vi "solar_target.vi"(11 "Target":string) -> ()   [LabVIEW 2018]
doc: "SOLAR target template."
uses:
  solar/solar.lvclass
  solar/solar Msg EnQ (This).vi
  solar/solar Msg UE Generate.vi
  voyager/solar_voy_def/solar_voy_def Import (Variants).vi
  solar/solar Msg Voyager (TLM).vi
panel:
  in  "data in":cluster{dbl}
  out "data out":cluster{dbl}
  out "Time":timestamp
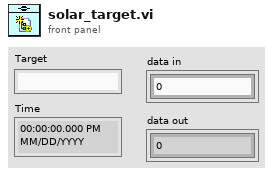
[diagram p1: front panel]
types:
  T1 = typedef "solar_voy_def_ctl PACKET.ctl" = cluster{"PACKET_ID":T2, "ENDIAN":enum8{"BIG", "LITTLE"}, "DESC":string, "HZRD":bool, "ITEMS":T3[], "NoExport":bool, "last_time":timestamp, "last_count":u32, "last_data":string}
  T2 = typedef "solar_voy_def_ctl PACKET_ID.ctl" = cluster{"ID":u16, "CMD":enum8{"CMD", "TLM"}, "TARGET":string, "PACKET":string}
  T3 = typedef "solar_voy_def_ctl ITEM.ctl" = cluster{"NAME":string, "OFFSET":i32, "SIZE":i32, "TYPE":T4, "EACH_SIZE":i32, "LVTYPE":T5, "MIN":dbl, "MAX":dbl, "DEFAULT":string, "DESC":string, "ID":bool, "MODIFIERS":variant, "last_value":variant}
  T4 = typedef "solar_voy_def_ctl ITEM TYPE.ctl" = enum8{"BLOCK", "INT", "UINT", "FLOAT", "STRING"}
  T5 = typedef "solar_type Item Type.ctl" = enum16{"NULL", "UNKNOWN", "CLUSTER", "I8", "I16", "I32", "I64", "U8", "U16", "U32", "U64", "U8_ENUM", "U16_ENUM", "U32_ENUM", "SGL", "DBL", "BOOLEAN", "STRING", "PATH", "VISA", "TAG", "TIME", "I8_1D", "I16_1D", "I32_1D", "I64_1D", "U8_1D", "U16_1D", "U32_1D", "U64_1D", "U8_ENUM_1D", "U16_ENUM_1D", "U32_ENUM_1D", "SGL_1D", "DBL_1D", "BOOLEAN_1D", "STRING_1D", "PATH_1D", "VISA_1D", "TAG_1D", "TIME_1D", "I8_2D", "I16_2D", "I32_2D", "I64_2D", "U8_2D", "U16_2D", "U32_2D", "U64_2D", "U8_ENUM_2D", "U16_ENUM_2D", "U32_ENUM_2D", "SGL_2D", "DBL_2D", "BOOLEAN_2D", "STRING_2D", "PATH_2D", "VISA_2D", "TAG_2D", "TIME_2D"}
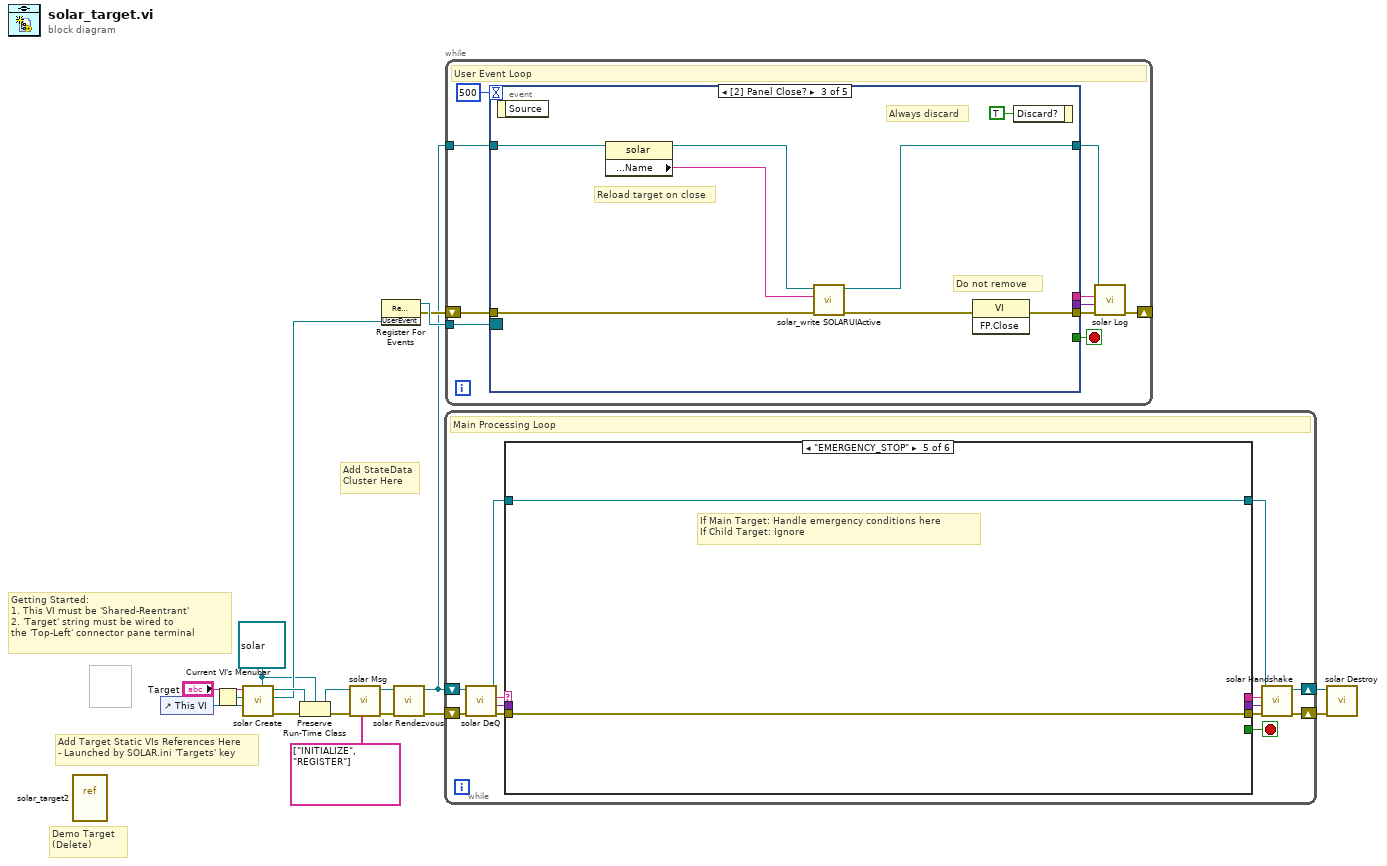
[diagram p0: block diagram]
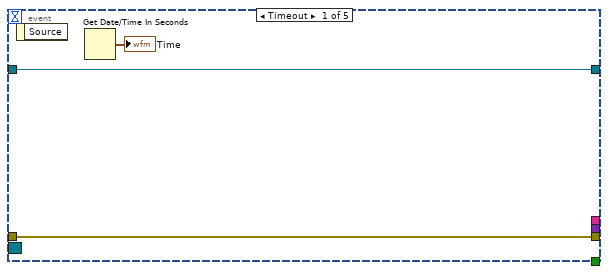
[diagram p2: hidden frame]
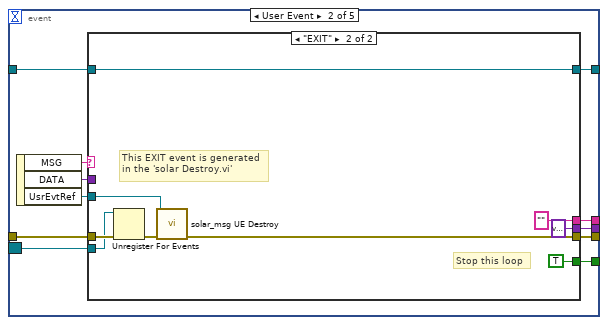
[diagram p3: hidden frame]
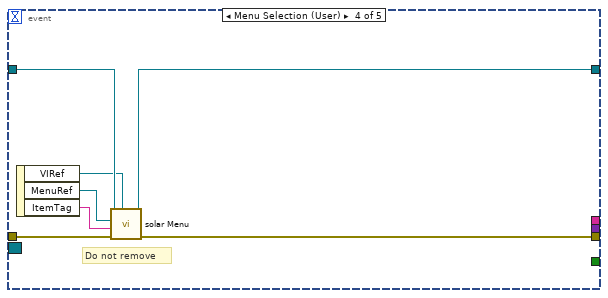
[diagram p5: hidden frame]
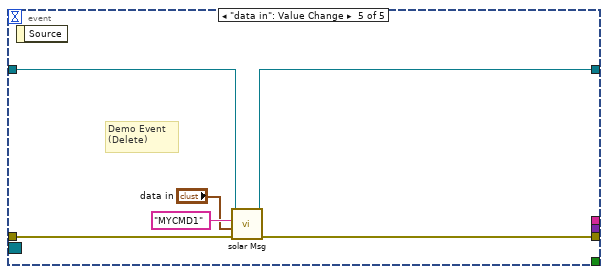
[diagram p6: hidden frame]
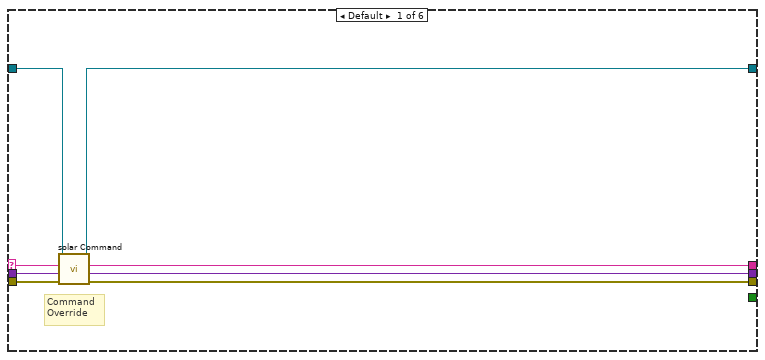
[diagram p7: hidden frame]
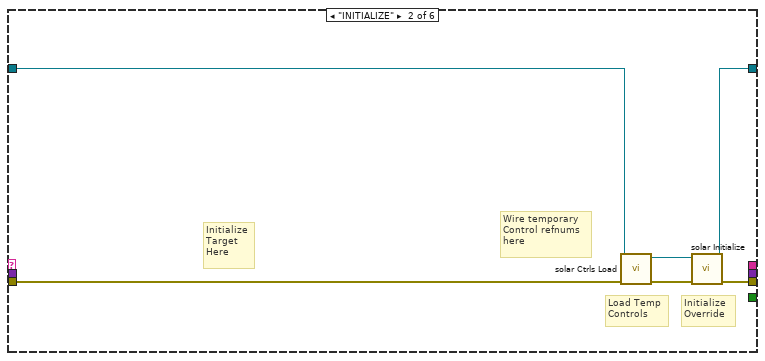
[diagram p8: hidden frame]
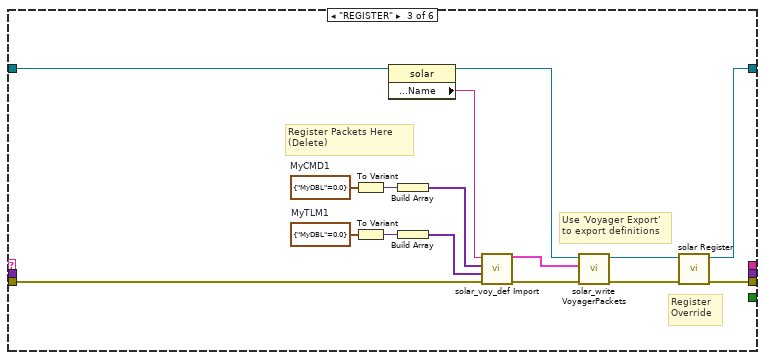
[diagram p9: hidden frame]
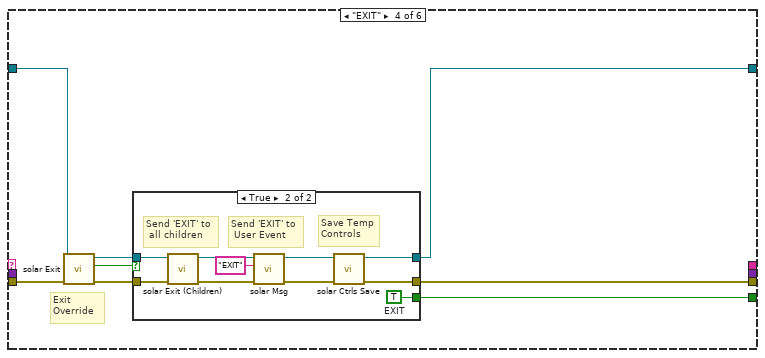
[diagram p10: hidden frame]
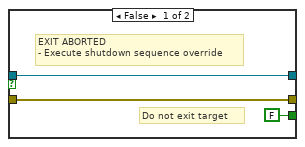
[diagram p11: hidden frame]
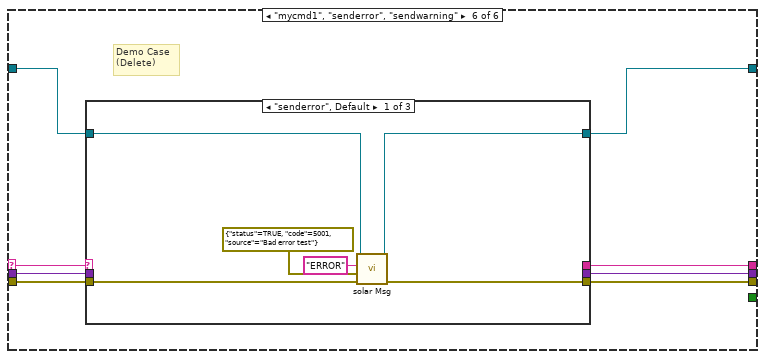
[diagram p12: hidden frame]
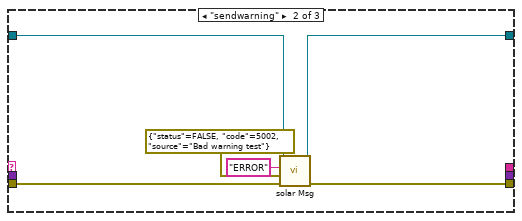
[diagram p13: hidden frame]
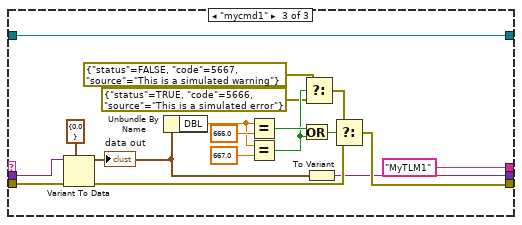
[diagram p14: hidden frame]
diagram:
  w11 = refnum<class "solar.lvclass"> refnum ("Default LVClass")
  # "Demo Target\n(Delete)"
  # "Getting Started:\n1. This VI must be 'Shared-Reentrant'\n2. 'Target' string must be wired to \nthe 'Top-Left' connector pane terminal"
  # "Add StateData\nCluster Here"
  # "Add Target Static VIs References Here\n- Launched by SOLAR.ini 'Targets' key"
  n1 = vi-ref "solar_target2.vi"() -> ()  [unwired: 1 out]
  n2 = control-ref of="This VI"() -> (w13:refnum<vi>)
  n3 = Current VI's Menubar() -> (w9:refnum<k9>)
  n4 = call "solar Create.vi"("Default LVClass"=w11, "VI Refnum"=w13, "VI MenuRef"=w9, "Target"="Target") -> ("error out"=w7:errorcluster, "UserEvent"=w14:refnum<user-event>, "solar"=w18:refnum<class "solar.lvclass">)  [unwired: 4 in, 1 out]
  n5 = Preserve Run-Time Class(object in=w18, error in=w7, 2:w11) -> (object out=w1:refnum<class "solar.lvclass">, error out=w3:errorcluster)
  n6 = call-poly "solar Msg.vi"("MSG Array"=string[] ["INITIALIZE", "REGISTER"] ("Script (\"PACKET{ITEM:VAL}\")"), "error in (no error)"=w3, "solar in"=w1) -> ("error out"=w6:errorcluster, "solar out"=w4:refnum<class "solar.lvclass">)  [unwired: 6 in, 1 out]
  n7 = register-events(w14) -> (reference out=w15:refnum<event-registration>, error out=w8:errorcluster)  [unwired: 2 in]
  n8 = call-dynamic "solar Rendezvous.vi"("error in (no error)"=w6, "solar in"=w4) -> ("error out"=w5:errorcluster, "solar out"=w2:refnum<class "solar.lvclass">)  [unwired: 6 in, 2 out]
  n9 = while {
    shift-right: [w28] -> w17
    shift-left: w5 -> [w30]
    shift-right: [w24] -> w16
    shift-left: w2 -> [w31]
    stop <- w23 stop-if-true
    # "Main Processing Loop"
    n10 = call "solar DeQ.vi"("error in (no error)"=w30, "solar in"=w31) -> ("error out"=w29:errorcluster, "DATA"=w19:variant, "MSG"=w20:string, "solar out"=w25:refnum<class "solar.lvclass">)  [unwired: 5 in, 1 out]
    n11 = case shown="\"EMERGENCY_STOP\"" w20 {
      selector: w20 -> [w34 _ _ _ _ w87]
      tunnel: [w39 w45 w52 w65 w83 w89] -> w27
      tunnel: w29 -> [w32 w41 w56 w69 w83 w92]
      tunnel: [w37 w44 w51 w64 w84 w85] -> w26
      tunnel: w25 -> [w38 w40 w57 w68 w84 w86]
      tunnel: w19 -> [w33 _ _ _ _ w90]
      tunnel: [_ _ _ w62 _ _] -> w23
      tunnel: [w36 _ _ _ _ w91] -> w22
      tunnel: [w35 _ _ _ _ w88] -> w21
      frame Default {
        # "Command\nOverride"
        n12 = call-dynamic "solar Command.vi"("error in (no error)"=w32, "CMD_DATA"=w33, "CMD"=w34, "solar in"=w38) -> ("error out"=w39:errorcluster, "TLM_DATA"=w35:variant, "TLM"=w36:string, "solar out"=w37:refnum<class "solar.lvclass">)  [unwired: 3 in, 1 out]
      }
      frame "INITIALIZE" {
        # "Wire temporary\nControl refnums\nhere"
        # "Load Temp\nControls"
        # "Initialize\nOverride"
        # "Initialize\nTarget\nHere"
        n13 = call "solar Ctrls Load.vi"("error in (no error)"=w41, "solar in"=w40) -> ("error out"=w43:errorcluster, "solar out"=w42:refnum<class "solar.lvclass">)  [unwired: 8 in]
        n14 = call-dynamic "solar Initialize.vi"("error in (no error)"=w43, "solar in"=w42) -> ("error out"=w45:errorcluster, "solar out"=w44:refnum<class "solar.lvclass">)  [unwired: 8 in]
      }
      frame "REGISTER" {
        w58 = cluster{"MyDBL":dbl} {"MyDBL"=0.0}  # MyTLM1
        w61 = cluster{"MyDBL":dbl} {"MyDBL"=0.0}  # MyCMD1
        # "Use 'Voyager Export'\nto export definitions"
        # "Register\nOverride"
        # "Register Packets Here\n(Delete)"
        n15 = To Variant(anything=w61) -> (Variant=w60:variant)
        n16 = To Variant(anything=w58) -> (Variant=w59:variant)
        n17 = property class="solar"(reference=w57) -> (reference out=w46:refnum<class "solar.lvclass">, "Accessors:This.Name"=w53:string)  [unwired: 1 in, 1 out]
        n18 = Build Array(w60) -> (w55:variant[])
        n19 = Build Array(w59) -> (w54:variant[])
        n20 = call-poly "solar_voy_def Import.vi"("error in (no error)"=w56, "TLMs"=w54, "CMDs"=w55, "TARGET"=w53) -> ("error out"=w48:errorcluster, "PACKETS"=w47:T1[])  [unwired: 6 in]
        n21 = call "solar_write VoyagerPackets.vi"("error in (no error)"=w48, "PACKETS"=w47, "solar in"=w46) -> ("error out"=w50:errorcluster, "solar out"=w49:refnum<class "solar.lvclass">)  [unwired: 7 in]
        n22 = call-dynamic "solar Register.vi"("error in (no error)"=w50, "solar in"=w49) -> ("error out"=w52:errorcluster, "solar out"=w51:refnum<class "solar.lvclass">)  [unwired: 8 in]
      }
      frame "EXIT" {
        # "Exit\nOverride"
        n23 = call-dynamic "solar Exit.vi"("error in (no error)"=w69, "solar in"=w68) -> ("error out"=w66:errorcluster, "Exit?"=w63:bool, "solar out"=w67:refnum<class "solar.lvclass">)  [unwired: 7 in]
        n24 = case shown="True" w63 {
          tunnel: w67 -> [w72 w77]
          tunnel: w66 -> [w71 w76]
          tunnel: [w71 w75] -> w65
          tunnel: [w72 w74] -> w64
          tunnel: [FALSE ("EXIT") w73] -> w62
          frame False {
            # "Do not exit target"
            # "EXIT ABORTED\n- Execute shutdown sequence override"
          }
          frame True {
            w73 = TRUE  # EXIT
            # "Save Temp\nControls"
            # "Send 'EXIT' to\n User Event"
            # "Send 'EXIT' to\n all children"
            n25 = call "solar Exit (Children).vi"("error in (no error)"=w76, "solar in"=w77) -> ("error out"=w79:errorcluster, "solar out"=w78:refnum<class "solar.lvclass">)  [unwired: 8 in]
            n26 = call-poly "solar Msg.vi"("error in (no error)"=w79, "MSG (last)"="EXIT" ("MSG (Last)"), "solar in"=w78) -> ("error out"=w81:errorcluster, "solar out"=w80:refnum<class "solar.lvclass">)  [unwired: 7 in]
            n27 = call "solar Ctrls Save.vi"("error in (no error)"=w81, "solar in"=w80) -> ("error out"=w75:errorcluster, "solar out"=w74:refnum<class "solar.lvclass">)  [unwired: 7 in, 1 out]
          }
        }
      }
      frame "EMERGENCY_STOP" {
        # "If Main Target: Handle emergency conditions here\nIf Child Target: Ignore"
      }
      frame "mycmd1", "senderror", "sendwarning" {
        # "Demo Case\n(Delete)"
        n28 = case shown="\"senderror\", Default" w87 {
          tunnel: w92 -> [w96 w102 w122]
          tunnel: [_ _ "MyTLM1" ("TLM")] -> w91
          tunnel: w90 -> [_ _ w120]
          tunnel: [w95 w101 w116] -> w89
          tunnel: [_ _ w106] -> w88
          tunnel: w86 -> [w94 w100 w105]
          tunnel: [w93 w99 w105] -> w85
          frame "senderror", Default {
            n29 = call-poly "solar Msg.vi"("error in (no error)"=w96, "TLM_DATA (No HDR)"=errorcluster {"status"=TRUE, "code"=5001, "source"="Bad error test"} ("t"), "TLM"="ERROR", "solar in"=w94) -> ("error out"=w95:errorcluster, "solar out"=w93:refnum<class "solar.lvclass">)  [unwired: 6 in]
          }
          frame "sendwarning" {
            n30 = call-poly "solar Msg.vi"("error in (no error)"=w102, "TLM_DATA (No HDR)"=errorcluster {"status"=FALSE, "code"=5002, "source"="Bad warning test"} ("t"), "TLM"="ERROR", "solar in"=w100) -> ("error out"=w101:errorcluster, "solar out"=w99:refnum<class "solar.lvclass">)  [unwired: 6 in]
          }
          frame "mycmd1" {
            n31 = Variant To Data(error in=w122, type=cluster{"DBL":dbl} {"DBL"=0.0}, Variant=w120) -> (data=w118:cluster{"DBL":dbl}, error out=w117:errorcluster)
            "data out" <- w118
            n32 = Unbundle By Name(w118) -> ("DBL"=w112:dbl)
            n33 = Equal?(x=w112, y=666.0) -> (x = y?=w114:bool)
            n34 = Equal?(x=w112, y=667.0) -> (x = y?=w110:bool)
            n35 = Or(x=w114, y=w110) -> (x .or. y?=w111:bool)
            n36 = Select(t=errorcluster {"status"=FALSE, "code"=5667, "source"="This is a simulated warning"}, s=w110, f=errorcluster {"status"=TRUE, "code"=5666, "source"="This is a simulated error"} ("t")) -> (s? t:f=w107:errorcluster)
            n37 = To Variant(anything=w118) -> (Variant=w106:variant)
            n38 = Select(t=w107, s=w111, f=w117) -> (s? t:f=w116:errorcluster)
          }
        }
      }
    }
    n39 = call "solar Handshake.vi"("error in (no error)"=w27, "TLM_DATA"=w21, "TLM"=w22, "solar in"=w26) -> ("error out"=w28:errorcluster, "solar out"=w24:refnum<class "solar.lvclass">)  [unwired: 6 in]
  }
  n40 = while {
    shift-right: [w126] -> _
    shift-left: w8 -> [w131]
    tunnel: w15 -> [w132]
    tunnel: w2 -> [w129]
    stop <- w130 stop-if-true
    # "User Event Loop"
    n41 = event shown="[2] Panel Close?" {
      selector: w132 -> [_ w143 _ _ _]
      dyn-events: _ -> [_ _ _ _ _]
      timeout: 500 -> [_ _ _ _ _]
      tunnel: w131 -> [w135 w144 w162 w172 w178]
      tunnel: [w135 w145 w164 w171 w177] -> w128
      tunnel: [_ w142 _ _ _] -> w130
      tunnel: w129 -> [w133 w137 w163 w168 w176]
      tunnel: [_ w140 _ _ _] -> w125
      tunnel: [w133 w138 w159 w167 w175] -> w127
      tunnel: [_ w136 _ _ _] -> w124
      event Timeout {
        n42 = event-data() -> ()  [unwired: 1 in, 1 out]
        n43 = Get Date/Time In Seconds() -> (seconds since 1Jan1904=→"Time":timestamp)
      }
      event User Event {
        n44 = event-data() -> ("MSG"=w146:string, "DATA"=w141:variant, "UsrEvtRef"=w139:refnum<user-event>)  [unwired: 1 in]
        n45 = case shown="\"EXIT\"" w146 {
          tunnel: [w148 w156] -> w145
          tunnel: w144 -> [w148 w157]
          tunnel: w143 -> [_ w153]
          tunnel: w139 -> [_ w155]
          tunnel: [_ TRUE] -> w142
          tunnel: w141 -> [_ _]
          tunnel: [_ ""] -> w140
          tunnel: [w147 w150] -> w138
          tunnel: w137 -> [w147 w150]
          tunnel: [_ variant] -> w136
          frame Default {
          }
          frame "EXIT" {
            # "Stop this loop"
            # "This EXIT event is generated\nin the 'solar Destroy.vi'"
            n46 = Unregister For Events(event registration refnum=w153, error in=w157) -> (error out=w154:errorcluster)
            n47 = call "solar_msg UE Destroy.vi"("error in (no error)"=w154, "UserEvent"=w155) -> ("error out"=w156:errorcluster)  [unwired: 9 in]
          }
        }
      }
      event Panel Close? {
        # "Do not remove"
        # "Reload target on close"
        # "Always discard"
        n48 = event-data() -> ()  [unwired: 1 in, 1 out]
        n49 = property class="solar"(reference=w163) -> (reference out=w160:refnum<class "solar.lvclass">, "Accessors:This.Name"=w158:string)  [unwired: 1 in, 1 out]
        n50 = call "solar_write SOLARUIActive.vi"("error in (no error)"=w162, "Target"=w158, "solar in"=w160) -> ("error out"=w161:errorcluster, "solar out"=w159:refnum<class "solar.lvclass">)  [unwired: 7 in]
        n51 = invoke class="VI" method="FP.Close"(error in=w161) -> (error out=w164:errorcluster)  [unwired: 2 in, 2 out]
        n52 = event-data("Discard?"=TRUE) -> ()  [unwired: 1 in, 1 out]
      }
      event Menu Selection (User) {
        # "Do not remove"
        n53 = event-data() -> ("VIRef"=w166:refnum<vi>, "MenuRef"=w169:refnum<k9>, "ItemTag"=w170:string)  [unwired: 1 in]
        n54 = call "solar Menu.vi"("VIRef"=w166, "error in (no error)"=w172, "ItemTag"=w170, "MenuRef"=w169, "solar in"=w168) -> ("error out"=w171:errorcluster, "solar out"=w167:refnum<class "solar.lvclass">)  [unwired: 5 in]
      }
      event "data in": Value Change {
        # "Demo Event\n(Delete)"
        n55 = event-data() -> ()  [unwired: 1 in, 1 out]
        n56 = call-poly "solar Msg.vi"("error in (no error)"=w178, "DATA (last)"="data in", "MSG (last)"="MYCMD1", "solar in"=w176) -> ("error out"=w177:errorcluster, "solar out"=w175:refnum<class "solar.lvclass">)  [unwired: 5 in, 1 out]
      }
    }
    n57 = call "solar Log.vi"("error in (no error)"=w128, "DATA"=w124, "MSG"=w125, "solar in"=w127) -> ("error out"=w126:errorcluster)  [unwired: 6 in, 1 out]
  }
  n58 = call "solar Destroy.vi"("error in (no error)"=w17, "solar in"=w16) -> ()  [unwired: 9 in, 1 out]
